vi "02passwordcoder-SIMPLEchanger.vi"() -> (0 "pass":string="0891", 1 "Boolean":bool, 2 "name":string="Admin")   [LabVIEW 2010]
panel:
  in  "Nombre":string
  in  "Password":string
  in  "CANC":bool
  in  "OK Button":bool
  # "INGRESE UN NUEVO\nNOMBRE DE USUARIO \nY CONTRASEÑA"
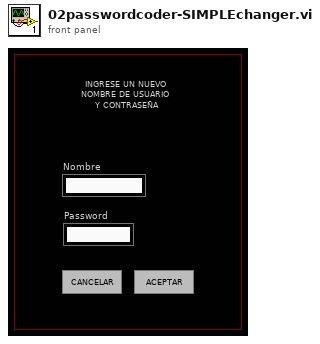
[diagram p1: front panel]
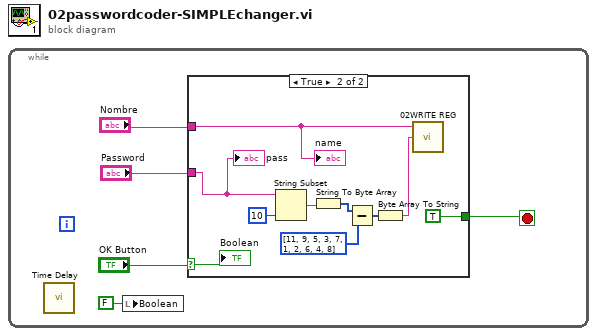
[diagram p0: block diagram]
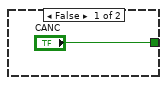
[diagram p2: hidden frame]
diagram:
  n1 = while {
    stop <- w1 stop-if-true
    n2 = call "Time Delay"() -> ()  [unwired: 11 in, 1 out]
    n3 = local write "Boolean"(FALSE ("Boolean")) -> ()
    n4 = case shown="True" "OK Button" {
      selector: "OK Button" -> [_ w7]
      tunnel: ["CANC" TRUE ("CANC")] -> w1
      tunnel: "Nombre" -> [_ w10]
      tunnel: "Password" -> [_ w8]
      frame False {
      }
      frame True {
        n5 = String Subset(string=w8, length (rest)=10 ("length (rest)")) -> (substring=w11:string)  [unwired: 1 in]
        n6 = String To Byte Array(string=w11) -> (unsigned byte array=w14:u8[])
        n7 = Subtract(x=w14, y=u8[] [11, 9, 5, 3, 7, 1, 2, 6, 4, 8]) -> (x-y=w15:u8[])
        n8 = Byte Array To String(unsigned byte array=w15) -> (string=w9:string)
        n9 = call "02WRITE REG.vi"("Password"=w9, "Nombre"=w10) -> ()  [unwired: 3 in]
        "name" <- w10
        "pass" <- w8
        "Boolean" <- w7
      }
    }
  }
